vi "Controller_ModuleQueue.vi"(7 "Enum":T1, 8 "error in (no error)":errorcluster, 11 "Data in":T2) -> (0 "error out":errorcluster, 1 "Queue size":i32, 2 "Data out":T2, 3 "queue out":refnum<queue>)   [LabVIEW 2020]
uses:
  #typedef_Controller_Data.ctl
  #typedef_Controller_States.ctl
  #typedef_ControllerQueue_States.ctl
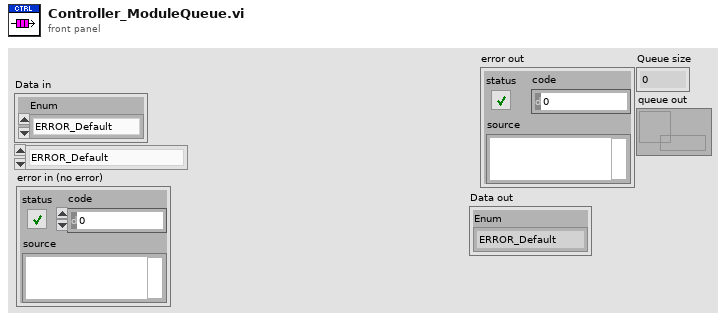
[diagram p1: front panel]
types:
  T1 = typedef "#typedef_ControllerQueue_States.ctl" = enum16{"ERROR_Default", "Obtain", "GetRef", "Enqueue", "EnqueueAtOpp", "GetStatus", "Flush", "Release"}
  T2 = typedef "#typedef_Controller_Data.ctl" = cluster{"Enum":T3}
  T3 = typedef "#typedef_Controller_States.ctl" = enum16{"ERROR_Default"}
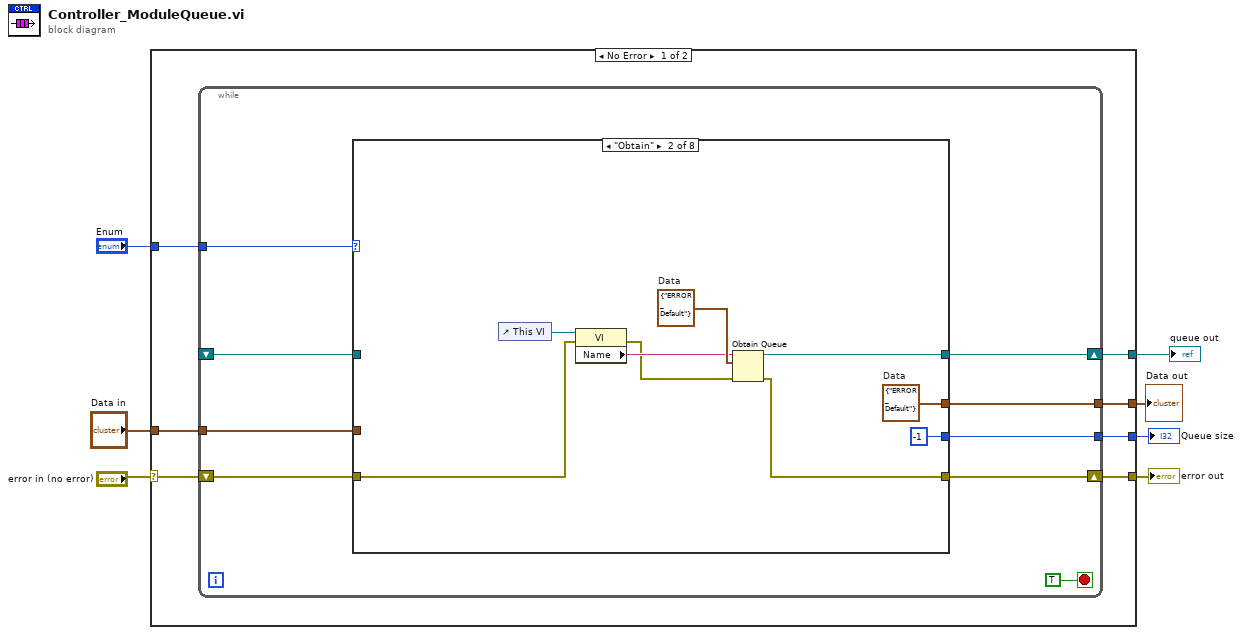
[diagram p0: block diagram]
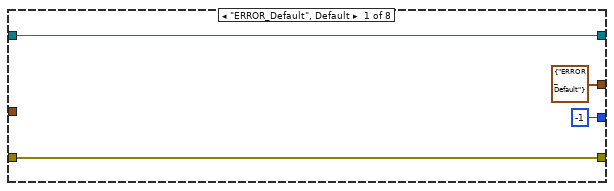
[diagram p2: hidden frame]
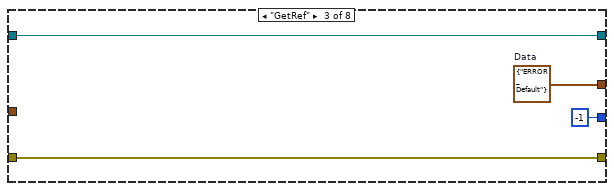
[diagram p3: hidden frame]
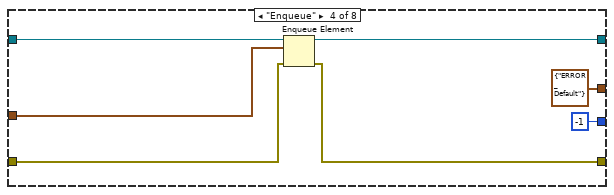
[diagram p4: hidden frame]
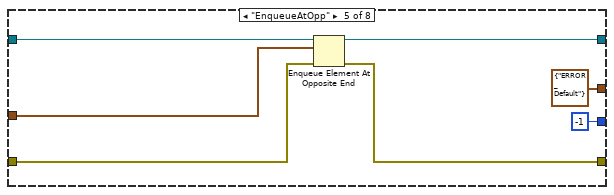
[diagram p5: hidden frame]
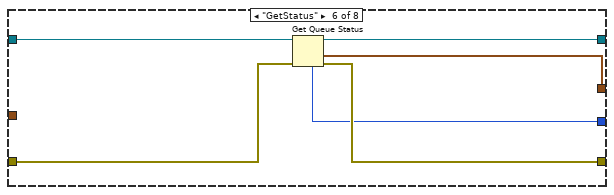
[diagram p6: hidden frame]
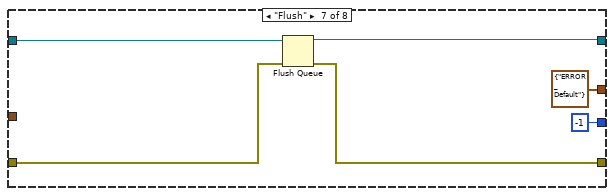
[diagram p7: hidden frame]
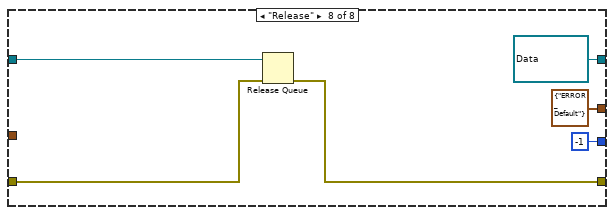
[diagram p8: hidden frame]
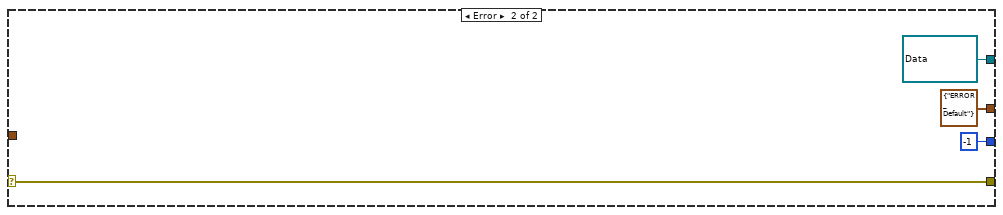
[diagram p9: hidden frame]
diagram:
  n1 = case shown="No Error" "error in (no error)" {
    selector: "error in (no error)" -> [w14 w76]
    tunnel: [w13 w76] -> w6
    tunnel: "Enum" -> [w12 _]
    tunnel: "Data in" -> [w11 _]
    tunnel: [w10 -1 ("# elements in queue")] -> w3
    tunnel: [w9 refnum<queue> refnum ("queue out")] -> w1
    tunnel: [w8 T2 {"Enum"=enum."ERROR_Default"} ("Data")] -> w2
    frame No Error {
      n2 = while {
        shift-right: [w22] -> w13
        shift-left: w14 -> [w23]
        tunnel: w12 -> [w21]
        tunnel: w11 -> [w20]
        tunnel: [w18] -> w10
        shift-right: [w17] -> w9
        shift-left: _ -> [w16]
        tunnel: [w15] -> w8
        stop <- TRUE stop-if-true
        n3 = case shown="\"Obtain\"" w21 {
          tunnel: w23 -> [w25 w29 w39 w44 w51 w58 w64 w71]
          tunnel: [w25 w35 w39 w45 w50 w57 w63 w70] -> w22
          tunnel: w20 -> [_ _ _ w43 w52 _ _ _]
          tunnel: [-1 ("# elements in queue") -1 -1 -1 -1 w56 -1 ("# elements in queue") -1 ("# elements in queue")] -> w18
          tunnel: [w27 w34 w38 w46 w53 w59 w65 refnum<queue> refnum ("queue out")] -> w17
          tunnel: w16 -> [w27 _ w38 w47 w54 w60 w66 w72]
          tunnel: [T2 {"Enum"=enum."ERROR_Default"} ("Data") w32 w37 T2 {"Enum"=enum."ERROR_Default"} ("Data") T2 {"Enum"=enum."ERROR_Default"} ("Data") w55 T2 {"Enum"=enum."ERROR_Default"} ("Data") T2 {"Enum"=enum."ERROR_Default"} ("Data")] -> w15
          frame "ERROR_Default", Default {
          }
          frame "Obtain" {
            w32 = T2 {"Enum"=enum."ERROR_Default"}  # Data
            w33 = T2 {"Enum"=enum."ERROR_Default"}  # Data
            n4 = control-ref of="This VI"() -> (w31:refnum<vi>)
            n5 = property class="VI"(reference=w31, error in=w29) -> (error out=w28:errorcluster, "Name"=w30:string)  [unwired: 1 out]
            n6 = Obtain Queue(name (unnamed)=w30, element data type=w33, error in (no error)=w28) -> (queue out=w34:refnum<queue>, error out=w35:errorcluster)  [unwired: 2 in, 1 out]
          }
          frame "GetRef" {
            w37 = T2 {"Enum"=enum."ERROR_Default"}  # Data
          }
          frame "Enqueue" {
            n7 = Enqueue Element(queue=w47, element=w43, error in (no error)=w44) -> (queue out=w46:refnum<queue>, error out=w45:errorcluster)  [unwired: 1 in, 1 out]
          }
          frame "EnqueueAtOpp" {
            n8 = Enqueue Element At Opposite End(queue=w54, element=w52, error in (no error)=w51) -> (queue out=w53:refnum<queue>, error out=w50:errorcluster)  [unwired: 1 in, 1 out]
          }
          frame "GetStatus" {
            n9 = Get Queue Status(queue=w60, error in (no error)=w58) -> (queue out=w59:refnum<queue>, error out=w57:errorcluster, # elements in queue=w56:i32, elements=w55:T2[])  [unwired: 1 in, 4 out]
          }
          frame "Flush" {
            n10 = Flush Queue(queue=w66, error in (no error)=w64) -> (queue out=w65:refnum<queue>, error out=w63:errorcluster)  [unwired: 1 out]
          }
          frame "Release" {
            n11 = Release Queue(queue=w72, error in (no error)=w71) -> (error out=w70:errorcluster)  [unwired: 1 in, 2 out]
          }
        }
      }
    }
    frame Error {
    }
  }
  "error out" <- w6
  "Queue size" <- w3
  "Data out" <- w2
  "queue out" <- w1
